vi "Apply APU Acceleration.vi"(9 "reset":bool, 10 "acceleration":fxp<+,18,-20>, 11 "desired speed":fxp<+/-,23,2>) -> (3 "actual speed":fxp<+/-,23,2>)   [LabVIEW 2013, in "Engine Simulation Toolkit.lvlib" / "APU.lvlib"]
uses:
  APU.lvlib
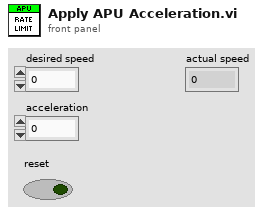
[diagram p1: front panel]
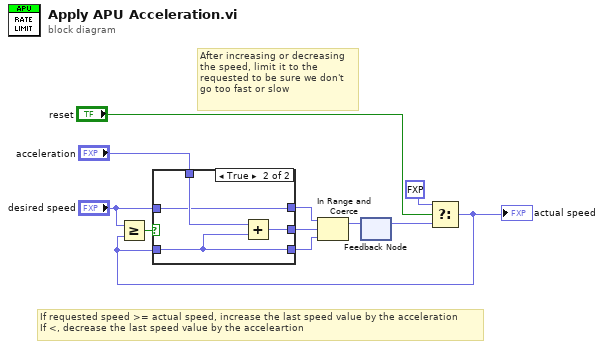
[diagram p0: block diagram]
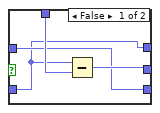
[diagram p2: hidden frame]
diagram:
  # "After increasing or decreasing the speed, limit it to the requested to be sure we don't go too fast or slow"
  # "If requested speed >= actual speed, increase the last speed value by the acceleration\nIf <, decrease the last speed value by the acceleartion"
  n1 = feedback #1() -> (w2:fxp<+/-,41,3>)  [unwired: 1 in]
  n2 = Select(t=fxp<+,1,1> 0.0, s="reset", f=w2) -> (s? t:f=w1:fxp<+/-,41,3>)
  "actual speed" <- w1
  n3 = Greater Or Equal?(x="desired speed", y=w1) -> (x >= y?=w9:bool)
  n4 = case shown="True" w9 {
    tunnel: w1 -> [w12 w16]
    tunnel: "acceleration" -> [w15 w19]
    tunnel: [w14 w18] -> w8
    tunnel: [w12 w17] -> w11
    tunnel: "desired speed" -> [w13 w17]
    tunnel: [w13 w16] -> w10
    frame False {
      n5 = Subtract(x=w12, y=w15) -> (x-y=w14:fxp<+/-,41,3>)
    }
    frame True {
      n6 = Add(x=w19, y=w16) -> (x+y=w18:fxp<+/-,41,3>)
    }
  }
  n7 = In Range and Coerce(upper limit=w11, x=w8, lower limit=w10) -> (coerced(x)=w3:fxp<+/-,41,3>)  [unwired: 1 out]
  n8 = feedback-in #1(w3) -> ()
